vi "inverseTransformCoords_3d.vi"(0 "x":dbl, 5 "y":dbl, 7 "z":dbl, 9 "current stage pos (px)":dbl[](array[numeric]), 11 "transform properties":T1={"theta (deg)"=0.0, "X sc factor (px/step)"=1.0, "Y sc factor (px/step)"=1.0, "zero loc (x,y,z)"=[0.0, 0.0], "flip y?"=FALSE, "flip x?"=FALSE, "gamma (deg)"=25.0, "flip z?"=FALSE, "Z sc factor (px/step)"=0.1098, "actuator"={"Actuator COM"="COM3", "Actuator type"=enum."Scientifica"}, "safe space (steps)"=[-69533, 0, -29190]} {"Y sc factor (px/step)" format="%#_13g"; "X sc factor (px/step)" format="%#_13g"; "theta (deg)" format="%#_13g"}) -> (4 "x out":dbl, 6 "y out":dbl, 10 "z out":dbl)   [LabVIEW 2015]
uses:
  <vilib>/Analysis/NI_AALPro.lvlib
  <vilib>/Analysis/coordinate.llb/2D Cartesian Coordinate Rotation (Scalar).vi
  pipette cleaning/pressure box/cleaning_soft/controls/actuator_type.ctl
  pipette cleaning/pressure box/cleaning_soft/controls/actuator_cluster.ctl
  transform_properties_actuators.ctl
panel:
  # "INVERSE"
  # "what kind\nregular: transform using the transform properties\ninverse: transform using the OPPOSITE of transform properties\n               ie if steps -> px is wired in, the transform will be px -> steps"
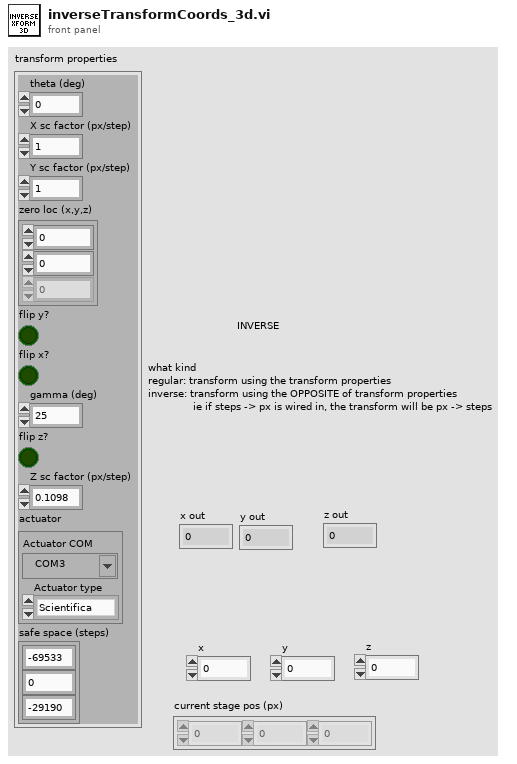
[diagram p1: front panel]
types:
  T1 = typedef "transform_properties_actuators.ctl" = cluster{"theta (deg)":dbl, "X sc factor (px/step)":dbl, "Y sc factor (px/step)":dbl, "zero loc (x,y,z)":dbl[], "flip y?":bool, "flip x?":bool, "gamma (deg)":dbl, "flip z?":bool, "Z sc factor (px/step)":dbl, "actuator":T2, "safe space (steps)":i32[]}
  T2 = typedef "actuator_cluster.ctl" = cluster{"Actuator COM":refnum<visa-resource-name>, "Actuator type":T3}
  T3 = typedef "actuator_type.ctl" = enum16{"Scientifica", "Sutter", "Demo", "Off"}
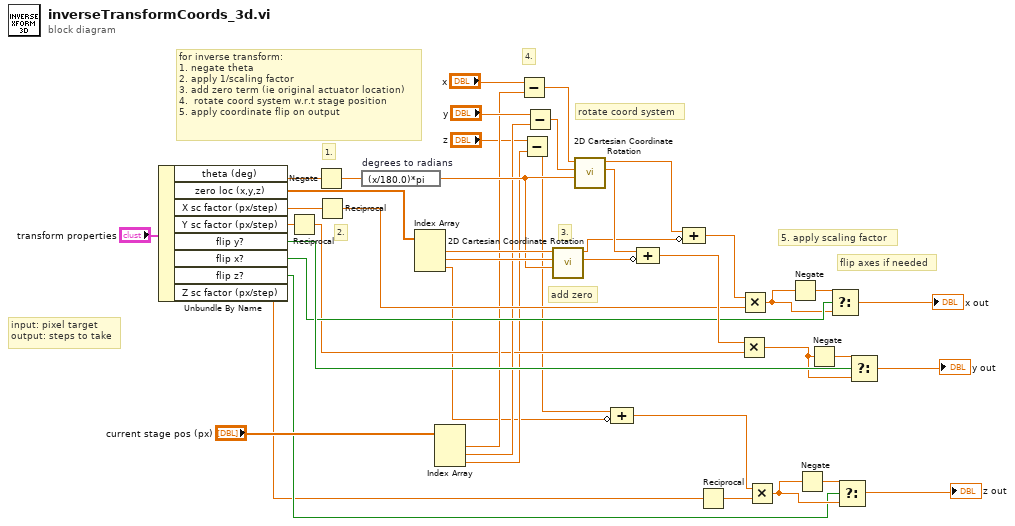
[diagram p0: block diagram]
diagram:
  # "4."
  # "3."
  # "2."
  # "1."
  # "input: pixel target\noutput: steps to take"
  # "add zero"
  # "for inverse transform:\n1. negate theta\n2. apply 1/scaling factor\n3. add zero term (ie original actuator location)\n4.  rotate coord system w.r.t stage position\n5. apply coordinate flip on output"
  # "flip axes if needed"
  # "5. apply scaling factor"
  # "rotate coord system"
  n1 = Unbundle By Name("transform properties") -> ("theta (deg)"=w37:dbl, "zero loc (x,y,z)"=w40:dbl[], "X sc factor (px/step)"=w36:dbl, "Y sc factor (px/step)"=w12:dbl, "flip y?"=w28:bool, "flip x?"=w25:bool, "flip z?"=w9:bool, "Z sc factor (px/step)"=w8:dbl)
  n2 = Reciprocal(x=w12) -> (1/x=w13:dbl)
  n3 = Negate(x=w37) -> (-x=w35:dbl)
  n4 = Reciprocal(x=w36) -> (1/x=w34:dbl)
  n5 = expression code="(x/180.0)*pi" "degrees to radians"(w35) -> (w22:dbl)
  n6 = Index Array(array=w40) -> (element #1=w33:dbl, element #2=w32:dbl, element #3=w2:dbl)  [unwired: 3 in]
  n7 = Index Array(array="current stage pos (px)") -> (element #1=w16:dbl, element #2=w14:dbl, element #3=w4:dbl)  [unwired: 3 in]
  n8 = Subtract(x="x", y=w16) -> (x-y=w18:dbl)
  n9 = Subtract(x="z", y=w4) -> (x-y=w3:dbl)
  n10 = Subtract(x="y", y=w14) -> (x-y=w19:dbl)
  n11 = call-poly <vilib>:"2D Cartesian Coordinate Rotation.vi"("theta"=w22, "y"=w32, "x"=w33) -> ("y out"=w31:dbl, "x out"=w30:dbl)  [unwired: 6 in, 1 out]
  n12 = call-poly <vilib>:"2D Cartesian Coordinate Rotation.vi"("theta"=w22, "y"=w19, "x"=w18) -> ("y out"=w42:dbl, "x out"=w41:dbl)  [unwired: 6 in, 1 out]
  n13 = Compound Arithmetic op=ADD(w3, invert w2) -> (w1:dbl)
  n14 = Compound Arithmetic op=ADD(w42, invert w31) -> (w38:dbl)
  n15 = Compound Arithmetic op=ADD(w41, invert w30) -> (w39:dbl)
  n16 = Reciprocal(x=w8) -> (1/x=w7:dbl)
  n17 = Multiply(x=w38, y=w13) -> (x*y=w27:dbl)
  n18 = Multiply(x=w39, y=w34) -> (x*y=w24:dbl)
  n19 = Multiply(x=w1, y=w7) -> (x*y=w10:dbl)
  n20 = Negate(x=w24) -> (-x=w26:dbl)
  n21 = Negate(x=w10) -> (-x=w11:dbl)
  n22 = Negate(x=w27) -> (-x=w29:dbl)
  n23 = Select(t=w26, s=w25, f=w24) -> (s? t:f=→"x out":dbl)
  n24 = Select(t=w11, s=w9, f=w10) -> (s? t:f=→"z out":dbl)
  n25 = Select(t=w29, s=w28, f=w27) -> (s? t:f=→"y out":dbl)
